vi "StringToDoubleArray.vi"(1 "String":string) -> (0 "MecTargets":dbl[](array[numeric]) caption="Predef. Positions" format="%.2f")   [LabVIEW 2012]
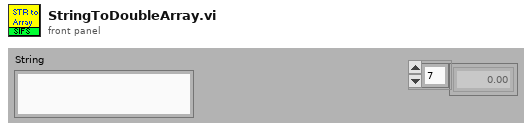
[diagram p1: front panel]
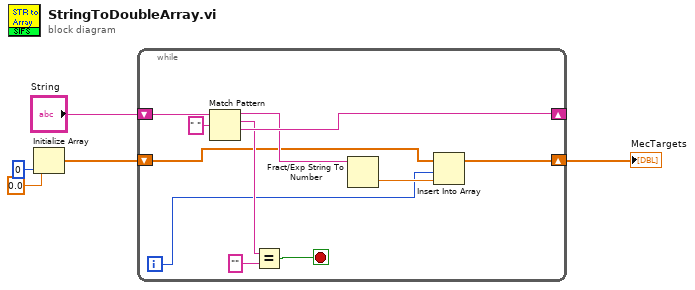
[diagram p0: block diagram]
diagram:
  n1 = Initialize Array(0.0 ("element"), 0 ("dimension size")) -> (w2:dbl[])
  n2 = while {
    shift-right: [w14] -> _
    shift-left: "String" -> [w16]
    shift-right: [w7] -> w1
    shift-left: w2 -> [w9]
    i -> [w8]
    stop <- w6 stop-if-true
    n3 = Match Pattern(string=w16, regular expression=" ") -> (before substring=w10:string, match substring=w13:string, after substring=w14:string)  [unwired: 2 out]
    n4 = Equal?(x=w13, y="") -> (x = y?=w6:bool)
    n5 = Fract/Exp String To Number(string=w10) -> (number=w11:dbl)  [unwired: 4 out]
    n6 = Insert Into Array(array=w9, index=w8, new element=w11) -> (w7:dbl[])
  }
  "MecTargets" <- w1
